vi "Get TSInstall by Version.vi"(8 "error in":errorcluster, 9 "Architecture":T2, 10 "Version":string, 11 "ITSDiscovery in":refnum<class "ITSDiscovery.lvclass">) -> (0 "error out":errorcluster, 3 "TSInstall Out":T1)   [LabVIEW 2025]
doc: "This VI retrieves a TestStand installation matching a specified version and architecture."
uses:
  ITSDiscovery/ITSDiscovery.lvclass
  Type Definitions/Architecture--enum.ctl
  Type Definitions/TSInstall--cluster.ctl
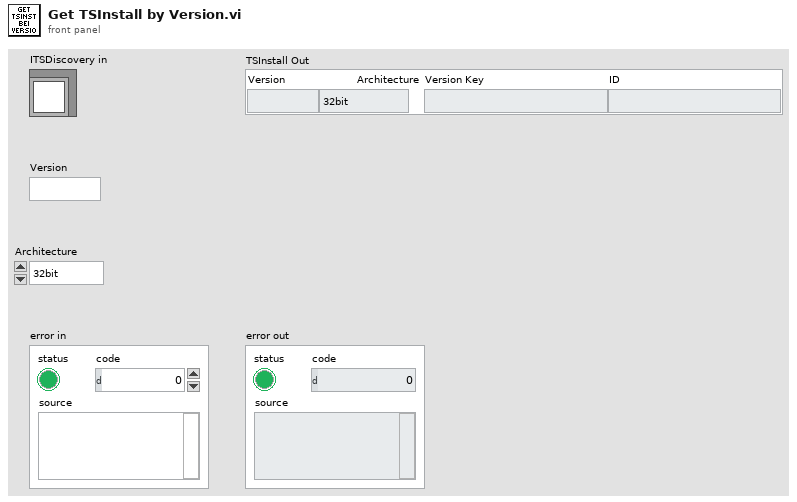
[diagram p1: front panel]
types:
  T1 = typedef "TSInstall--cluster.ctl" = cluster{"Version":string, "Architecture":T2, "Version Key":string, "ID":string}
  T2 = typedef "Architecture--enum.ctl" = enum16{"32bit", "64bit"}
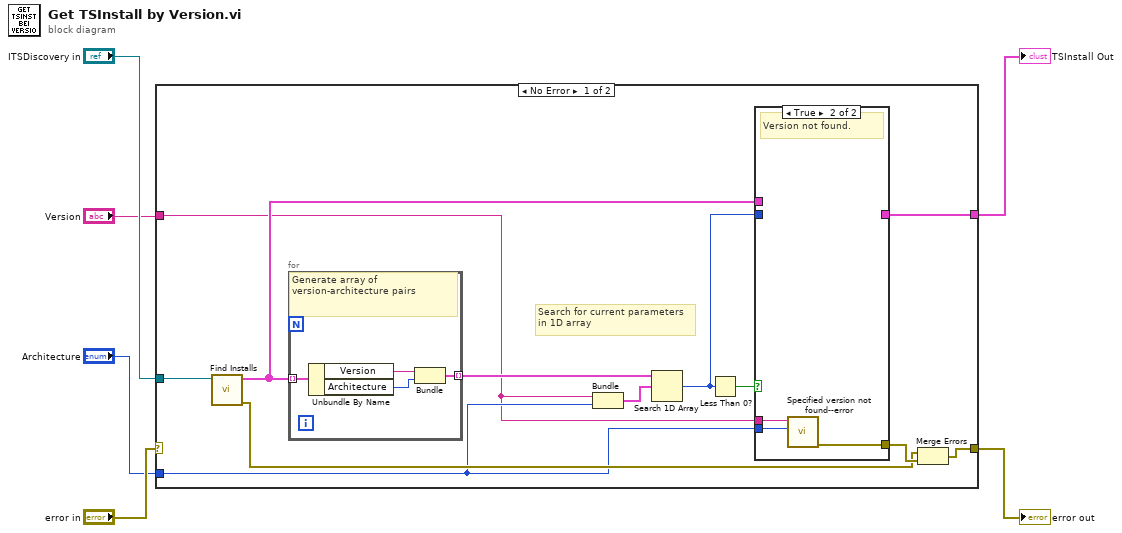
[diagram p0: block diagram]
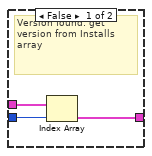
[diagram p2: hidden frame]
diagram:
  n1 = case shown="No Error" "error in" {
    selector: "error in" -> [_ w29]
    tunnel: "ITSDiscovery in" -> [w15 _]
    tunnel: [w16 w29] -> w5
    tunnel: [w9 _] -> w3
    tunnel: "Architecture" -> [w8 _]
    tunnel: "Version" -> [w7 _]
    frame No Error {
      # "Search for current parameters\nin 1D array"
      n2 = call-dynamic "Find Installs.vi"("ITSDiscovery in"=w15) -> ("error out"=w17:errorcluster, "TSInstalls Out"=w11:T1[])  [unwired: 9 in]
      n3 = for {
        tunnel: w11 -> [w28] mode=indexing
        tunnel: [w25] -> w14 mode=indexing
        # "Generate array of version-architecture pairs"
        n4 = Unbundle By Name(w28) -> ("Version"=w27:string, "Architecture"=w26:T2)
        n5 = Bundle("Version"=w27, "Architecture"=w26) -> (w25:cluster{"Version":string, "Architecture":T2})  [unwired: 1 in]
      }
      n6 = Bundle("Version"=w7, "Architecture"=w8) -> (w13:cluster{"Version":string, "Architecture":T2})  [unwired: 1 in]
      n7 = Search 1D Array(1D array=w14, element=w13) -> (index of element=w10:i32)  [unwired: 1 in]
      n8 = Less Than 0?(x=w10) -> (x < 0?=w12:bool)
      n9 = case shown="True" w12 {
        tunnel: w7 -> [_ w23]
        tunnel: w8 -> [_ w22]
        tunnel: w11 -> [w21 _]
        tunnel: w10 -> [w20 _]
        tunnel: [w19 _] -> w9
        tunnel: [_ w24] -> w18
        frame False {
          # "Version found: get version from Installs array"
          n10 = Index Array(array=w21, index=w20) -> (element=w19:T1)
        }
        frame True {
          # "Version not found."
          n11 = call "Specified version not found--error.vi"("Architecture"=w22, "Version"=w23) -> ("error out"=w24:errorcluster)  [unwired: 9 in]
        }
      }
      n12 = Merge Errors(w17, w18) -> (w16:errorcluster)
    }
    frame Error {
      # "Pass error without further action"
    }
  }
  "error out" <- w5
  "TSInstall Out" <- w3
